vi "CreateGetVersionSerializableData.vi"(0 "LVClassLibrary Ref":refnum<vi>, 5 "Application":refnum<vi>, 7 "SerializableData_v2.ctl path":path, 9 "Mutate_v2_to_v3.vi path":path, 11 "error in (no error)":errorcluster, 12 "Template VI path":path, 13 "SaveTo Path":path) -> (4 "LVClassLibrary Ref":refnum<vi>, 6 "Application":refnum<vi>, 15 "error out":errorcluster)   [LabVIEW 2019, in "BlueSerializationScripts.lvlib"]
uses:
  BlueSerializationScripts.lvlib
  BlueSerialVirtualFolders.ctl
  44a6fcf3-7c1c-47d8-bcb4-0ef1b2cf7892.vi
  5295cb97-9c40-4f97-af7b-c4055edc2ab1.vi
  <vilib>/Utility/error.llb/Clear Errors.vi
  <userlib>/_OpenG.lib/file/file.llb/File Exists - Scalar__ogtk.vi
  BlueSerialProviderGlobal.vi
  <vilib>/Utility/traverseref.llb/Traverse for GObjects.vi
  BlueUtilityScripts/RefIsOwner.vi
  BlueUtilityScripts/BlueUtilityScripts.lvlib
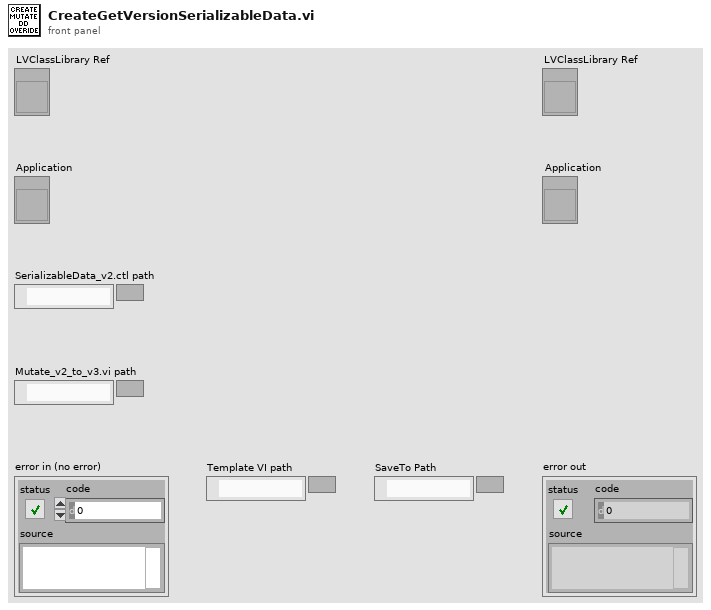
[diagram p1: front panel]
types:
  T1 = enum32{"invalid scope", "public", "private", "protected", "community"}
  T2 = typedef "BlueSerializationScripts.lvlib/BlueSerialVirtualFolders.ctl" = enum16{"BlueSerialization", "Mutations"}
  T3 = enum32{"invalid VI type", "Standard VI", "Control VI", "Global VI", "Polymorphic VI", "Configuration VI", "SubSystem", "Facade VI", "Method VI"}
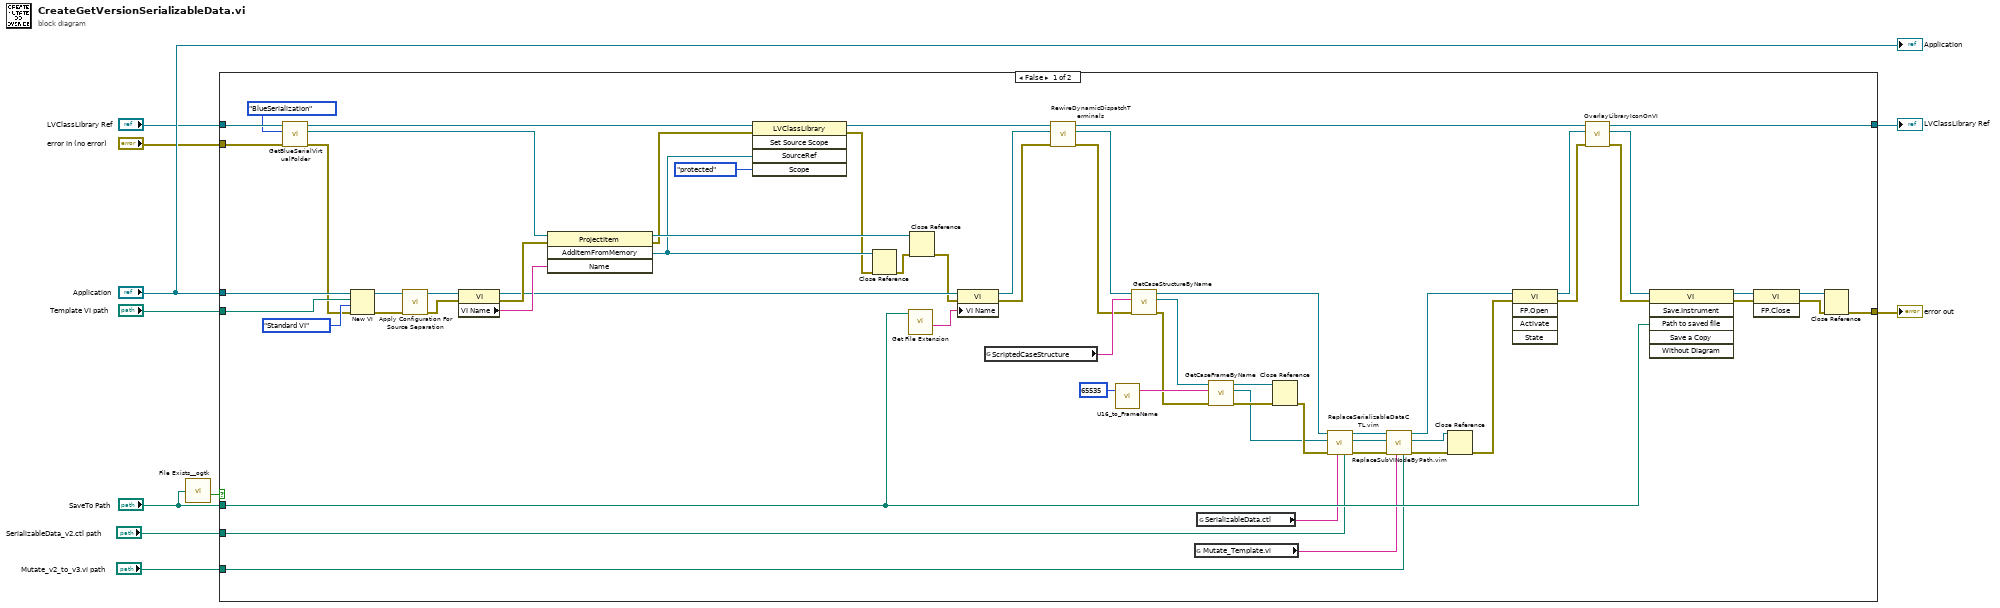
[diagram p0: block diagram]
diagram:
  n1 = call-poly <userlib>:"File Exists__ogtk.vi"("file path"="SaveTo Path") -> ("exists"=w2:bool)  [unwired: 6 in, 1 out]
  n2 = case shown="False" w2 {
    tunnel: "Application" -> [w72 _]
    tunnel: "Template VI path" -> [w71 _]
    tunnel: "error in (no error)" -> [w50 w73]
    tunnel: "LVClassLibrary Ref" -> [w51 w74]
    tunnel: "SerializableData_v2.ctl path" -> [w35 _]
    tunnel: [w21 w74] -> w5
    tunnel: [w65 w73] -> w4
    tunnel: "SaveTo Path" -> [w52 _]
    tunnel: "Mutate_v2_to_v3.vi path" -> [w26 _]
    frame False {
      n3 = call "GetBlueSerialVirtualFolder.vi"("error in (no error)"=w50, "Virtual Folder"=BlueSerialVirtualFolders."BlueSerialization", "LVClassLibrary Ref"=w51) -> ("error out"=w48:errorcluster, "Folder Refnum out"=w47:refnum<vi>, "LVClassLibrary Ref"=w15:refnum<vi>)  [unwired: 6 in]
      n4 = New VI(8:w48, 9:T3."Standard VI" ("vi type (standard vi)"), 10:w71, 11:w72) -> (0:w55:errorcluster, 3:w56:refnum<vi>)  [unwired: 3 out]
      n5 = call <vilib>:"Apply Configuration For Source Separation.vi"("error in (no error)"=w55, "VI in"=w56) -> ("error out"=w59:errorcluster, "VI out"=w61:refnum<vi>)  [unwired: 8 in]
      n6 = property class="VI"(reference=w61, error in=w59) -> (reference out=w62:refnum<vi>, error out=w64:errorcluster, "VI Name"=w63:string)
      n7 = invoke class="ProjectItem" method="AddItemFromMemory"(reference=w47, error in=w64, "Name"=w63) -> (reference out=w57:refnum<vi>, error out=w13:errorcluster, "AddItemFromMemory"=w12:refnum<vi>)  [unwired: 1 in, 1 out]
      n8 = invoke class="LVClassLibrary" method="Set Source Scope"(reference=w15, error in=w13, "SourceRef"=w12, "Scope"=T1."protected" ("scope")) -> (reference out=w14:refnum<vi>, error out=w11:errorcluster)  [unwired: 1 in, 3 out]
      n9 = Close Reference(reference=w12, error in (no error)=w11) -> (error out=w53:errorcluster)
      n10 = call <vilib>:"Get File Extension.vi"("file"=w52) -> ("filename without extension"=w60:string)  [unwired: 6 in, 4 out]
      n11 = Close Reference(reference=w57, error in (no error)=w53) -> (error out=w58:errorcluster)
      n12 = property class="VI"(reference=w62, error in=w58, "VI Name"=w60) -> (reference out=w46:refnum<vi>, error out=w45:errorcluster)
      n13 = global read "BlueSerialProviderGlobal.vi" "ScriptedCaseStructure"() -> (w44:string)
      n14 = call "RewireDynamicDispatchTerminals.vi"("error in (no error)"=w45, "VI Reference"=w46, "LVClassLibrary"=w14) -> ("error out"=w40:errorcluster, "VI Reference"=w43:refnum<vi>, "LVClassLibrary"=w22:refnum<vi>)  [unwired: 6 in]
      n15 = call "U16_to_FrameName.vi"("u16"=u16 65535) -> ("FrameName"=w41:string)  [unwired: 2 in]
      n16 = call "GetCaseStructureByName.vi"("error in (no error)"=w40, "CaseStructureLabel.Text"=w44, "VI Refnum"=w43) -> ("error out"=w39:errorcluster, "CaseStructure Ref"=w42:refnum<vi>, "VI Refnum"=w31:refnum<vi>)  [unwired: 6 in]
      n17 = global read "BlueSerialProviderGlobal.vi" "Mutate_Template.vi"() -> (w27:string)
      n18 = global read "BlueSerialProviderGlobal.vi" "SerializableData.ctl"() -> (w34:string)
      n19 = call "GetCaseFrameByName.vi"("error in (no error)"=w39, "FrameName"=w41, "CaseStructure Ref"=w42) -> ("error out"=w38:errorcluster, "Frame Ref"=w32:refnum<vi>, "CaseStructure Ref"=w37:refnum<vi>)  [unwired: 6 in]
      n20 = Close Reference(reference=w37, error in (no error)=w38) -> (error out=w33:errorcluster)
      n21 = call "ReplaceSerializableDataCTL.vim"("CTL path"=w35, "TypedefPath Name"=w34, "error in (no error)"=w33, "Owner"=w32, "VI Refnum"=w31) -> ("error out"=w28:errorcluster, "dup Owner"=w29:refnum<vi>, "dup VI Refnum"=w30:refnum<vi>)  [unwired: 4 in]
      n22 = call "ReplaceSubVINodeByPath.vim"("SubVI  path"=w26, "SubVI File Name"=w27, "error in (no error)"=w28, "Owner"=w29, "VI Refnum"=w30) -> ("error out"=w23:errorcluster, "dup Owner"=w24:refnum<vi>, "dup VI Refnum"=w25:refnum<vi>)  [unwired: 4 in]
      n23 = Close Reference(reference=w24, error in (no error)=w23) -> (error out=w36:errorcluster)
      n24 = invoke class="VI" method="FP.Open"(reference=w25, error in=w36) -> (reference out=w20:refnum<vi>, error out=w19:errorcluster)  [unwired: 3 in, 3 out]
      n25 = call "OverlayLibraryIconOnVI.vi"("error in (no error)"=w19, "VI Refnum out"=w20, "LVClassLibrary"=w22) -> ("error out"=w18:errorcluster, "VI Refnum out"=w17:refnum<vi>, "LVClassLibrary"=w21:refnum<vi>)  [unwired: 5 in, 1 out]
      n26 = invoke class="VI" method="Save.Instrument"(reference=w17, error in=w18, "Path to saved file"=w52) -> (reference out=w70:refnum<vi>, error out=w69:errorcluster)  [unwired: 3 in, 4 out]
      n27 = invoke class="VI" method="FP.Close"(reference=w70, error in=w69) -> (reference out=w67:refnum<vi>, error out=w66:errorcluster)  [unwired: 1 in, 1 out]
      n28 = Close Reference(reference=w67, error in (no error)=w66) -> (error out=w65:errorcluster)
    }
    frame True {
    }
  }
  "error out" <- w4
  "LVClassLibrary Ref" <- w5
  "Application" <- "Application"
